vi "global variable-骰子比大小獲勝次數.vi"() -> ()   [LabVIEW 2014]
panel:
  out "骰子比大小獲勝次數":i32
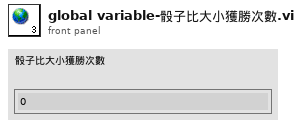
[diagram p1: front panel]
diagram:
